vi "Database Recordset Get Item From Fields.vi"(8 "error in (no error)":errorcluster caption="错误输入（无错误）", 10 "Index":i32, 11 "Database Recordset 输入":refnum<class "Database Recordset.lvclass"> caption="DNL_LabVIEW Object in") -> (0 "error out":errorcluster caption="错误输出", 2 "Item":refnum<k7>, 3 "Database Recordset 输出":refnum<class "Database Recordset.lvclass"> caption="DNL_LabVIEW Object out")   [LabVIEW 2011, in "Database Recordset.lvclass"]
uses:
  Database Recordset.lvclass
  Database Recordset.lvclass/Database Recordset.ctl
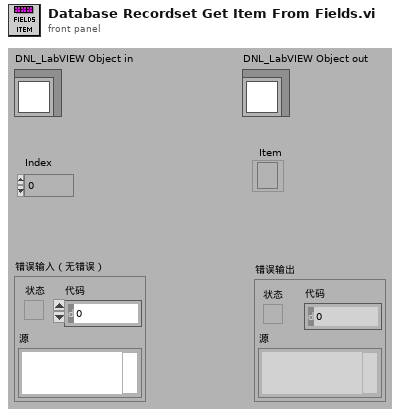
[diagram p1: front panel]
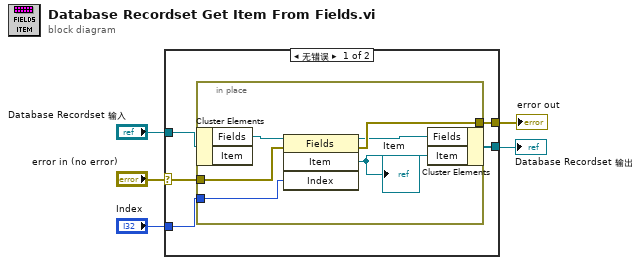
[diagram p0: block diagram]
diagram:
  n1 = case shown="无错误" "error in (no error)" {
    selector: "error in (no error)" -> [w10 w18]
    tunnel: [w9 w18] -> w4
    tunnel: [w6 w17] -> w2
    tunnel: "Database Recordset 输入" -> [w7 w17]
    tunnel: "Index" -> [w8 _]
    frame No Error {
      n2 = in-place {
        in-place-border: w10 -> [w16]
        in-place-border: [w15] -> w9
        in-place-border: w8 -> [w14]
        n3 = in-place-cluster #1(w7) -> ("Fields"=w13:refnum<k7>)  [unwired: 1 out]
        n4 = invoke class="Fields" method="Item"(reference=w13, error in=w16, "Index"=w14) -> (reference out=w12:refnum<k7>, error out=w15:errorcluster, "Item"=w11:refnum<k7>)  [unwired: 1 in, 1 out]
        "Item" <- w11
        n5 = in-place-cluster #1("Fields"=w12, "Item"=w11) -> (w6:refnum<class "Database Recordset.lvclass">)
      }
    }
    frame Error {
    }
  }
  "error out" <- w4
  "Database Recordset 输出" <- w2
